vi "Levelmeter.vi"(1 "Action":T4=enum."Identify", 2 "Parameters":variant) -> (6 "Output":variant, 7 "Stop":bool)   [LabVIEW 2024]
uses:
  Sub Controls/Instrument Actions.ctl
  Sub Controls/Public.ctl
  Sub Controls/Instrument Match.ctl
  Sub Controls/Factory Reset.ctl
  Sub Controls/Scan Output.ctl
  Sub Controls/Instrument IDN.ctl
  Sub Controls/User Event Command.ctl
  <vilib>/Instr/_visa.llb/VISA GPIB Control REN Mode.ctl
panel:
  in  "Factory Reset":T1
  out "Title":string="Levelmeter"
  in  "VISA resource name":refnum<visa-resource-name>
  in  "Instruments":T2[](array[typedef])=[{"Model"="LM-500", "Manufacturer"="Cryomagnetics", "Term Character"="", "Wait Time (mS)"=0, "Wait for SRQ"=FALSE, "Type"="Levelmeter"}]
  out "Model":string
  in  "Address":u16(ring)
  in  "Channel":bool
  in  "Public":T3
  out "Measurement":dbl[](array[numeric]) format="%^.3e"
  # "Ch. 2"
  # "Ch. 1"
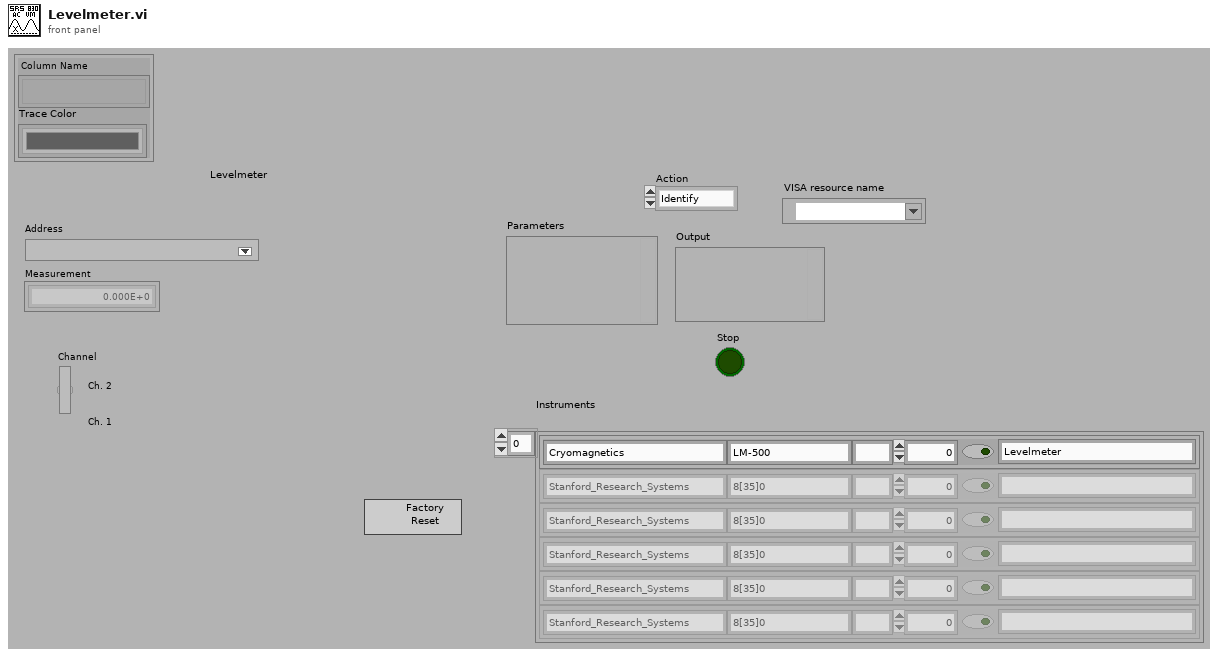
[diagram p1: front panel]
types:
  T1 = typedef "Factory Reset.ctl" = bool
  T2 = typedef "Instrument Match.ctl" = cluster{"Model":string, "Manufacturer":string, "Term Character":string, "Wait Time (mS)":u32, "Wait for SRQ":bool, "Type":string}
  T3 = typedef "Public.ctl" = cluster{"Column Name":string[], "Trace Color":u32[]}
  T4 = typedef "Instrument Actions.ctl" = enum16{"Scan", "Identify", "New", "Configure", "Initialize", "Test", "Read", "Close"}
  T5 = typedef "Scan Output.ctl" = cluster{"Manufacturer":string, "Model":string, "Info":string, "Revision":string, "error out":errorcluster}
  T6 = typedef "Instrument IDN.ctl" = cluster{"VISA Address":string, "Status":u16, "Manufacturer":string, "Model":string, "Info":string, "Info 2":string, "Misc Data":variant}
  T7 = typedef "User Event Command.ctl" = enum32{"Stop Config"}
  T8 = typedef "VISA GPIB Control REN Mode.ctl" = u16
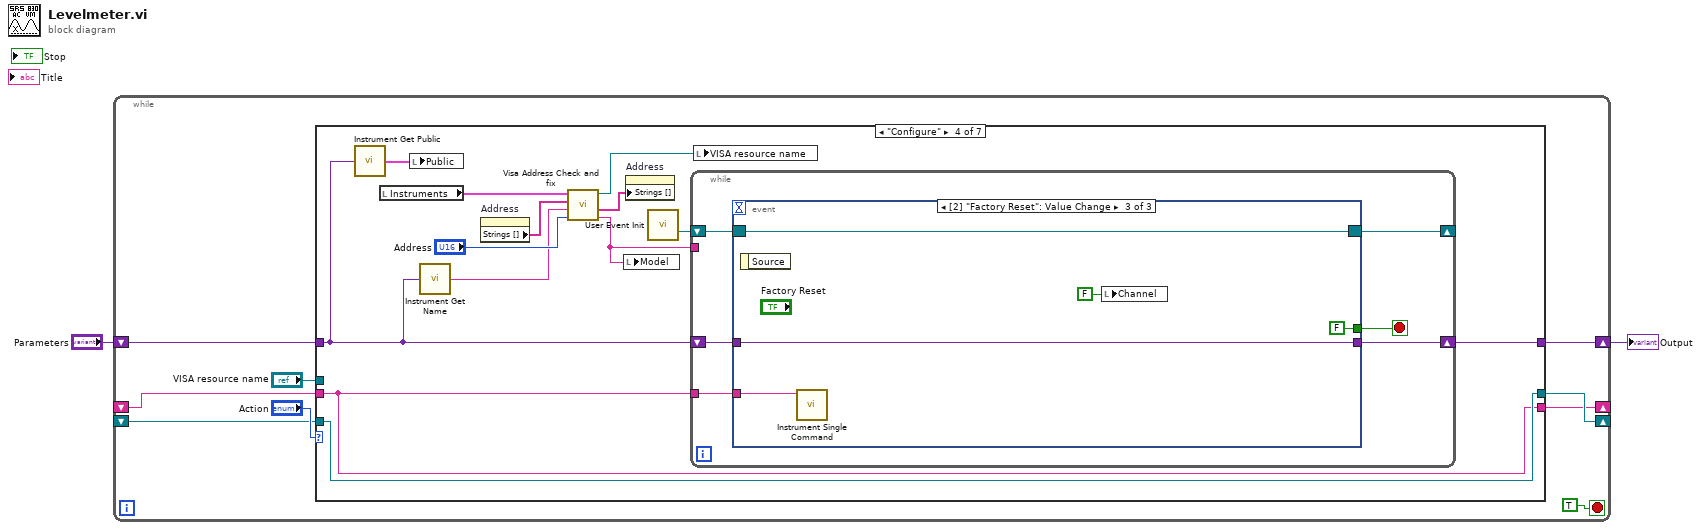
[diagram p0: block diagram]
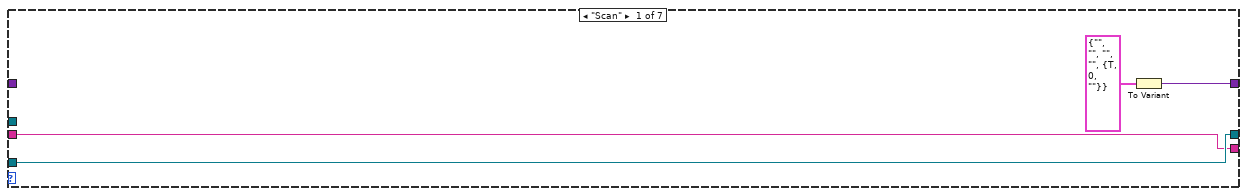
[diagram p2: hidden frame]
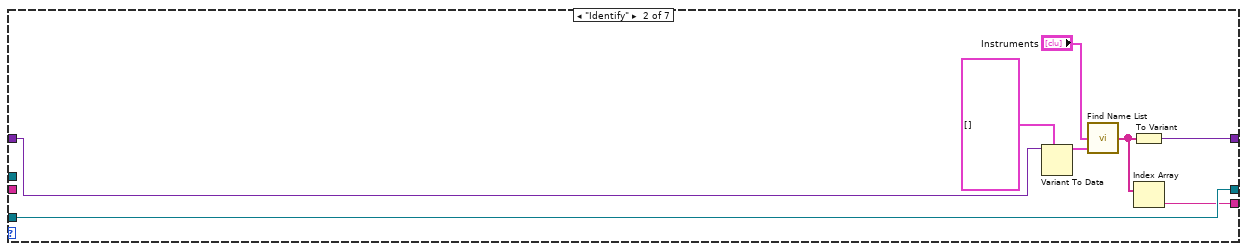
[diagram p3: hidden frame]
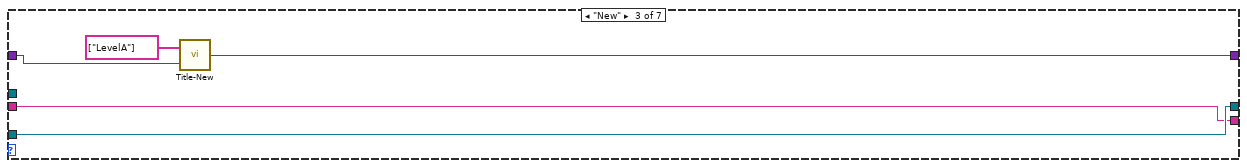
[diagram p4: hidden frame]
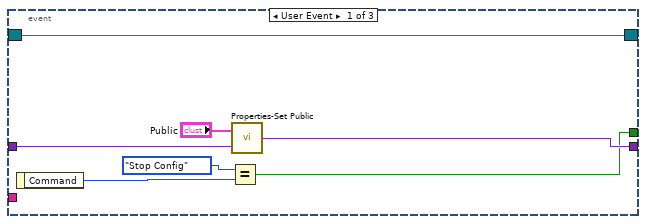
[diagram p5: hidden frame]
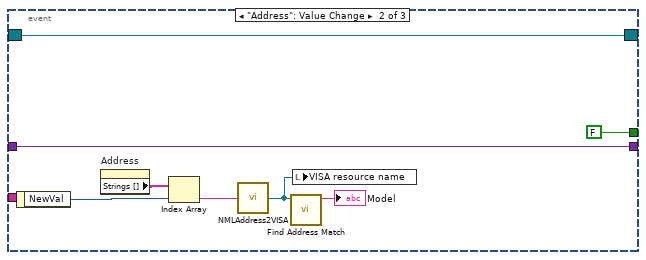
[diagram p6: hidden frame]
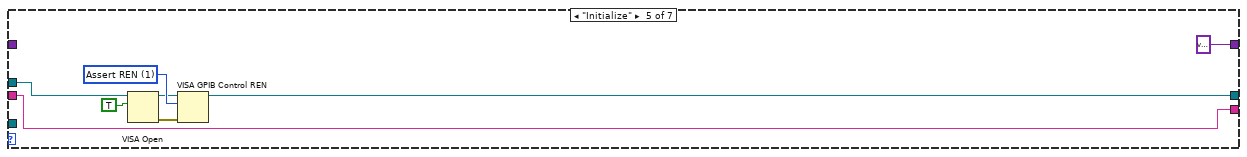
[diagram p7: hidden frame]
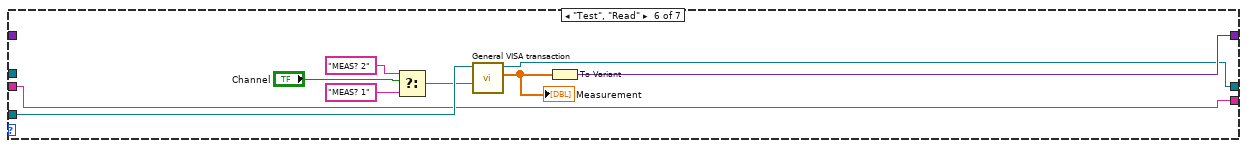
[diagram p8: hidden frame]
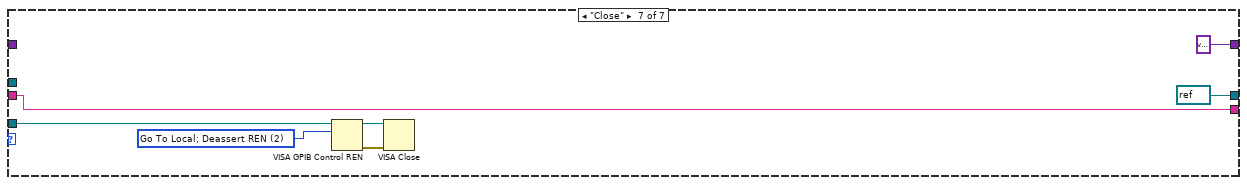
[diagram p9: hidden frame]
diagram:
  n1 = while {
    shift-right: [w10] -> _
    shift-left: _ -> [w9]
    shift-right: [w7] -> w1
    shift-left: "Parameters" -> [w8]
    shift-right: [w4] -> _
    shift-left: _ -> [w3]
    stop <- TRUE stop-if-true
    n2 = case shown="\"Configure\"" "Action" {
      tunnel: [w14 w23 w27 w41 w70 w83 refnum<visa-resource-name> refnum ("Open VISA Resource name")] -> w10
      tunnel: w9 -> [w14 w23 w27 w41 _ w82 w86]
      tunnel: w8 -> [_ w20 w28 w31 _ _ _]
      tunnel: [w13 w22 w25 w40 variant ("Variant") w84 variant ("Variant")] -> w7
      tunnel: "VISA resource name" -> [_ _ _ _ w69 _ _]
      tunnel: [w12 w16 w24 w29 w68 w80 w85] -> w4
      tunnel: w3 -> [w12 _ w24 w29 w68 w80 w85]
      frame "Scan" {
        n3 = To Variant(anything=T5 {"Manufacturer"="", "Model"="", "Info"="", "Revision"="", "error out"={"status"=TRUE, "code"=0, "source"=""}} ("Scan Output")) -> (Variant=w13:variant)
      }
      frame "Identify" {
        n4 = Variant To Data(type=T6[] [], Variant=w20) -> (data=w18:T6[])  [unwired: 1 in, 1 out]
        n5 = call "Find Name List.vi"("Bus Scan"=w18, "Instruments"="Instruments") -> ("Names"=w17:string[])  [unwired: 1 in]
        n6 = To Variant(anything=w17) -> (Variant=w22:variant)
        n7 = Index Array(array=w17) -> (element=w16:string)  [unwired: 1 in]
      }
      frame "New" {
        n8 = call "Title-New.vi"("Parameters"=w28, "Array"=string[] ["LevelA"]) -> ("Instrument Prop"=w25:variant)
      }
      frame "Configure" {
        n9 = call "Instrument Get Public.vi"("Variant"=w31) -> ("Public"=w39:T3)
        n10 = local read "Instruments"() -> (w30:T2[])
        n11 = local write "Public"(w39) -> ()
        n12 = call "Instrument Get Name.vi"("Parameters"=w31) -> ("Type"=w32:string)
        n13 = property on="Address" class="Ring (strict)"() -> ("Strings []"=w36:string[])  [unwired: 2 in, 2 out]
        n14 = call "Visa Address Check and fix.vi"("Address"="Address", "Name"=w32, "NML Addresses"=w36, "Instruments"=w30) -> ("Model"=w33:string, "NML Addresses"=w34:string[], "VISA resource name"=w35:refnum<visa-resource-name>)  [unwired: 3 out]
        n15 = local write "Model"(w33) -> ()
        n16 = property on="Address" class="Ring (strict)"("Strings []"=w34) -> ()  [unwired: 2 in, 2 out]
        n17 = call "User Event Init.vi"() -> ("Event Registration Refnum"=w38:refnum<event-registration>)  [unwired: 14 in, 1 out]
        n18 = while {
          shift-right: [w47] -> w40
          shift-left: w31 -> [w46]
          shift-right: [w43] -> _
          shift-left: w38 -> [w44]
          tunnel: w33 -> [_]
          tunnel: w29 -> [w42]
          stop <- w45 stop-if-true
          n19 = event shown="[2] \"Factory Reset\": Value Change" {
            selector: w44 -> [w48 w62 w67]
            dyn-events: [w48 w62 w67] -> w43
            timeout: _ -> [_ _ _]
            tunnel: [w50 FALSE FALSE] -> w45
            tunnel: w46 -> [w53 w56 w66]
            tunnel: [w54 w56 w66] -> w47
            tunnel: w42 -> [_ _ w64]
            event User Event {
              n20 = event-data() -> ("Command"=w52:T7)  [unwired: 1 in]
              n21 = Equal?(x=User_Event_Command."Stop Config", y=w52) -> (x = y?=w50:bool)
              n22 = call "Properties-Set Public.vi"("Variant"=w53, "New Public"="Public") -> ("Variant 2"=w54:variant)
            }
            event "Address": Value Change {
              n23 = event-data() -> ("NewVal"=w60:u16)  [unwired: 1 in]
              n24 = property on="Address" class="Ring (strict)"() -> ("Strings []"=w59:string[])  [unwired: 2 in, 2 out]
              n25 = Index Array(array=w59, index=w60) -> (element=w58:string)
              n26 = call "NMLAddress2VISA.vi"("NML Address"=w58) -> ("VISA resource name"=w55:refnum<visa-resource-name>)
              n27 = call "Find Address Match.vi"("VISA resource name"=w55) -> ("Model"=→"Model":string)  [unwired: 3 in, 3 out]
              n28 = local write "VISA resource name"(w55) -> ()
            }
            event Value Change {
              n29 = event-data() -> ()  [unwired: 1 in, 1 out]
              n30 = call "Instrument Single Command.vi"("VISA Name"=w64) -> ()  [unwired: 10 in, 1 out]
              n31 = local write "Channel"(FALSE ("Channel")) -> ()
            }
          }
        }
        n32 = local write "VISA resource name"(w35) -> ()
      }
      frame "Initialize" {
        w74 = T8 1 items=["Deassert REN", "Assert REN", "Go To Local; Deassert REN ", "Assert REN; Address Device", "Local Lockout (Addressed Devices)", "Local Lockout (This Device)", "Go To Local"] ("Mode")
        n33 = VISA Open(duplicate session (F)=TRUE, VISA resource name=w69) -> (VISA resource name=w72:refnum<visa-resource-name>, error out=w73:errorcluster)  [unwired: 3 in]
        n34 = VISA GPIB Control REN(8:w73, 10:w74, 11:w72) -> (3:w70:refnum<visa-resource-name>)  [unwired: 1 out]
      }
      frame "Test", "Read" {
        n35 = Select(t="MEAS? 2", s="Channel", f="MEAS? 1") -> (s? t:f=w78:string)
        n36 = call "General VISA transaction.vi"("Command String"=w78, "VISA Session"=w82) -> ("Measurement"=w81:dbl[], "dup VISA Session"=w83:refnum<visa-resource-name>)  [unwired: 4 in, 4 out]
        "Measurement" <- w81
        n37 = To Variant(anything=w81) -> (Variant=w84:variant)
      }
      frame "Close" {
        w90 = T8 2 items=["Deassert REN", "Assert REN", "Go To Local; Deassert REN ", "Assert REN; Address Device", "Local Lockout (Addressed Devices)", "Local Lockout (This Device)", "Go To Local"] ("Mode")
        n38 = VISA GPIB Control REN(10:w90, 11:w86) -> (0:w89:errorcluster, 3:w88:refnum<visa-resource-name>)  [unwired: 1 in]
        n39 = VISA Close(VISA resource name=w88, error in (no error)=w89) -> ()  [unwired: 1 out]
      }
    }
  }
  "Output" <- w1
